vi "QueryGrating.vi"(8 "error in (no error)":errorcluster, 11 "HRS_Spectrometer in":refnum<class "HRS_Spectrometer.lvclass">) -> (0 "error out":errorcluster, 3 "HRS_Spectrometer out":refnum<class "HRS_Spectrometer.lvclass">)   [LabVIEW 2023, in "HRS_Spectrometer.lvlib" / "HRS_Spectrometer.lvclass"]
uses:
  HRS_Spectrometer.lvclass
  HRS_Spectrometer.lvclass/HRS_Spectrometer.ctl
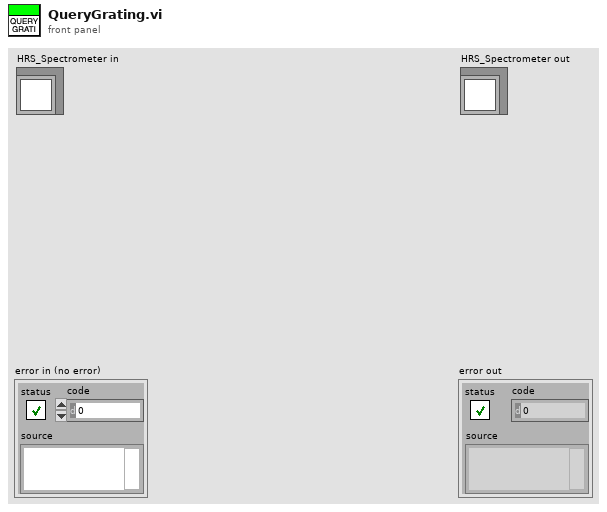
[diagram p1: front panel]
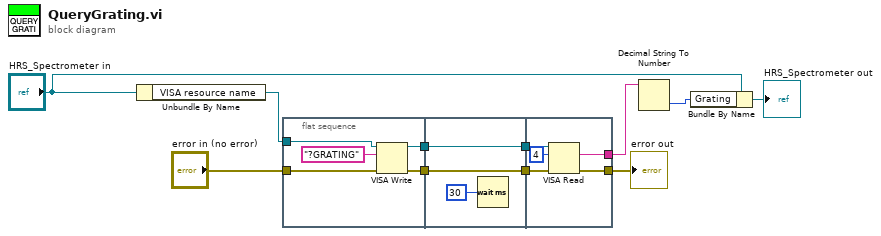
[diagram p0: block diagram]
diagram:
  n1 = Unbundle By Name("HRS_Spectrometer in") -> ("VISA resource name"=w4:refnum<visa-resource-name>)
  n2 = flat-sequence {
    tunnel: [w15] -> w11
    tunnel: [w14] -> w10
    tunnel: w4 -> [w13]
    tunnel: "error in (no error)" -> [w12]
    tunnel: w11 -> [w19]
    tunnel: w10 -> [w18]
    tunnel: [w19] -> w9
    tunnel: [w18] -> w8
    tunnel: w9 -> [w23]
    tunnel: w8 -> [w24]
    tunnel: [w22] -> w7
    tunnel: [w21] -> w2
    frame #0 {
      n3 = VISA Write(VISA resource name=w13, write buffer="?GRATING", error in (no error)=w12) -> (VISA resource name out=w15:refnum<visa-resource-name>, error out=w14:errorcluster)  [unwired: 1 out]
    }
    frame #1 {
      n4 = Wait (ms)(milliseconds to wait=u32 30) -> ()  [unwired: 1 out]
    }
    frame #2 {
      n5 = VISA Read(VISA resource name=w23, byte count=u32 4, error in (no error)=w24) -> (read buffer=w22:string, error out=w21:errorcluster)  [unwired: 2 out]
    }
  }
  n6 = Decimal String To Number(string=w7) -> (number=w1:i32)  [unwired: 2 in, 1 out]
  n7 = Bundle By Name(cluster="HRS_Spectrometer in", "Grating"=w1) -> (→"HRS_Spectrometer out":refnum<class "HRS_Spectrometer.lvclass">)
  "error out" <- w2
